vi "OSU_Sample.vi"() -> ()   [LabVIEW 2017]
uses:
  C:/Users/Ssantec_Test/Documents/Instrument_DLL_Sample_Labview_20220902_Ver1.2.2/DLL/x86/InstrumentDLL.dll
  DLL/x86/InstrumentDLL.dll
panel:
  in  "cmbdevname":u16(ring) caption="device name"
  in  "cmbosu_usb":u16(ring) caption="USB Resource"
  in  "txtPort":string caption="Port number(LAN)"
  in  "Address(GPIB、LAN)":string
  in  "OSU-110":T1(radio)
  in  "Target":enum32{"rdo100", "rdo110"}(radio)
  out "OSU":refnum<k24>
  in  "btn_Switch":bool
  in  "channel":u16(ring) items=["", "Ch1", "Ch2", "Ch3", "Ch4"]
  in  "Btn_DisConnect":bool
  in  "Btn_Connect":bool
  # "1. Connect"
  # "Communication"
  # "OSU-110"
  # "OSU-100"
  # "2. Setting function"
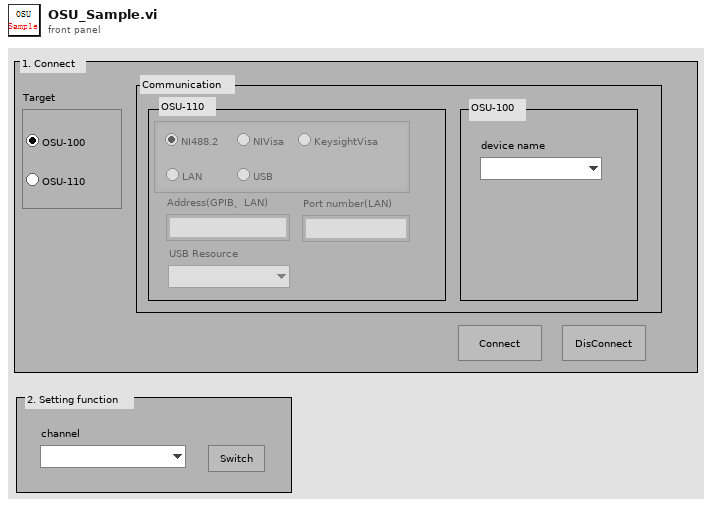
[diagram p1: front panel]
types:
  T1 = enum32{"rdiNI488", "rdiNIvisa", "rdikysightvisa", "rdoLAN", "rdiUSB"}
  T2 = enum8{"Enabled", "Disabled", "Disabled and Grayed Out"}
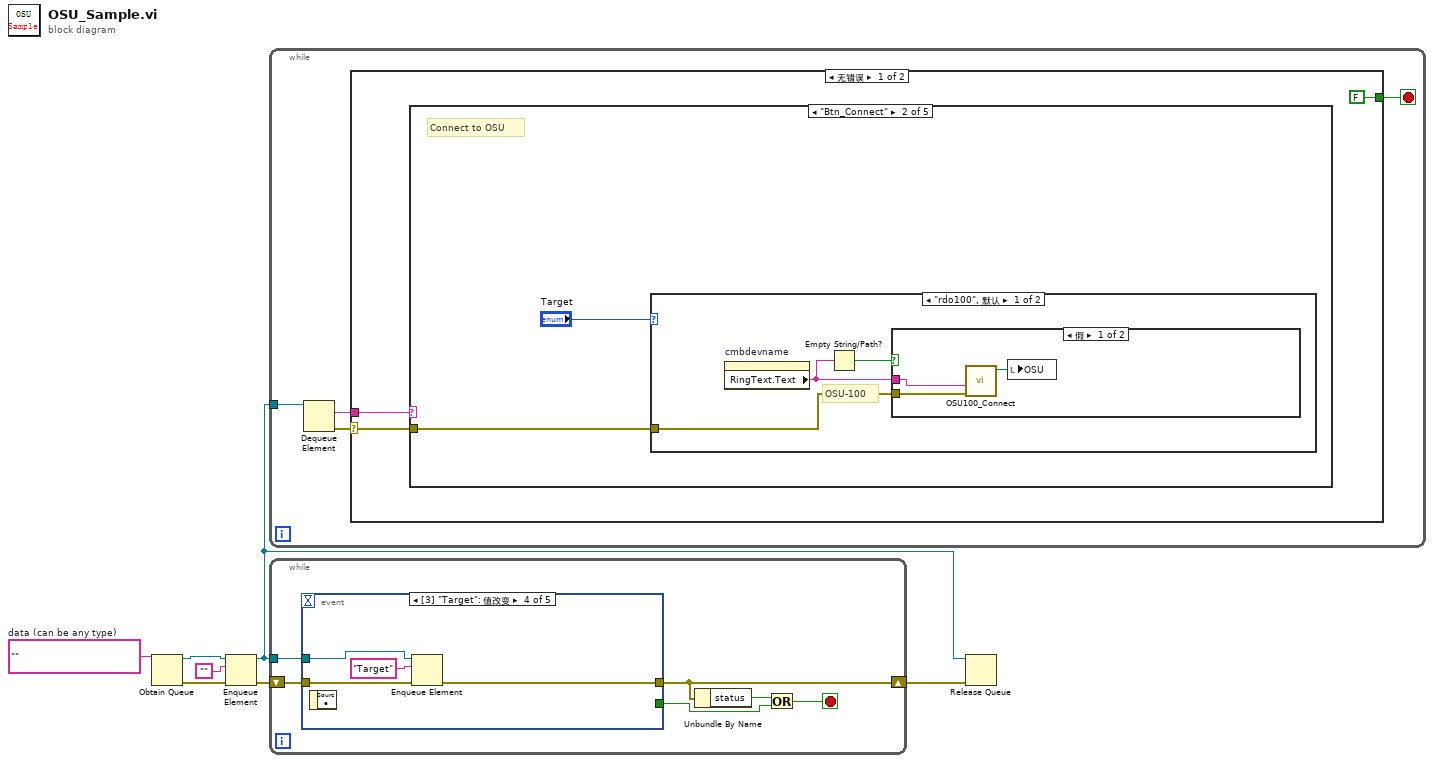
[diagram p0: block diagram]
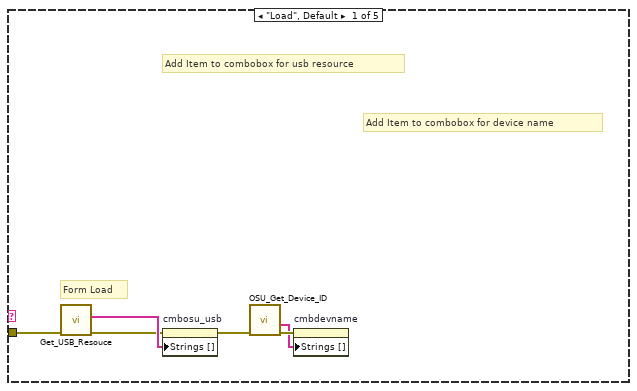
[diagram p2: hidden frame]
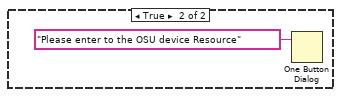
[diagram p3: hidden frame]
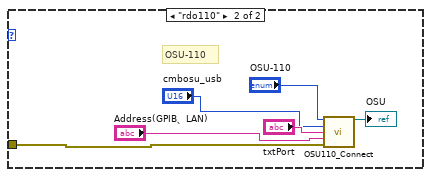
[diagram p4: hidden frame]
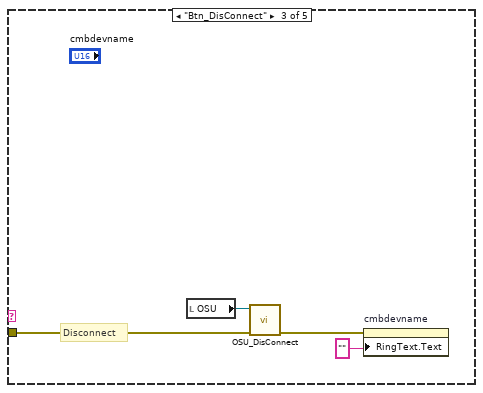
[diagram p5: hidden frame]
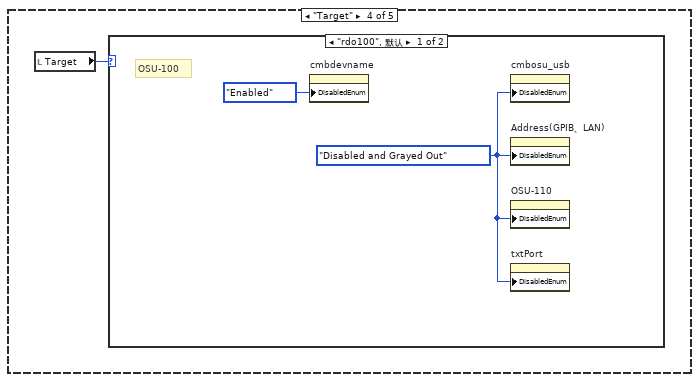
[diagram p6: hidden frame]
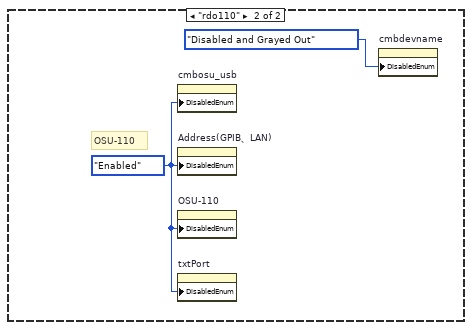
[diagram p7: hidden frame]
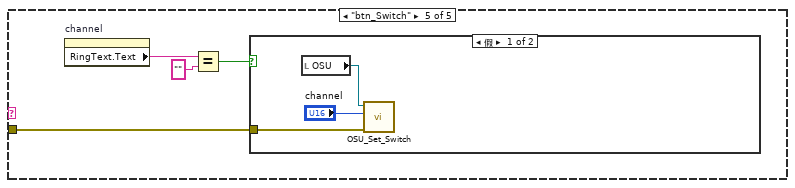
[diagram p8: hidden frame]
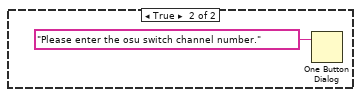
[diagram p9: hidden frame]
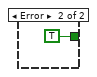
[diagram p10: hidden frame]
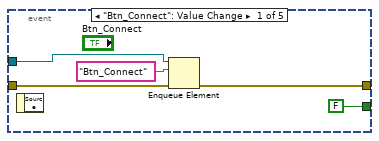
[diagram p11: hidden frame]
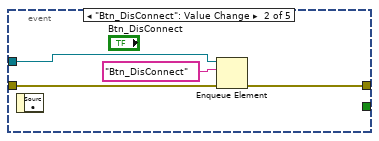
[diagram p12: hidden frame]
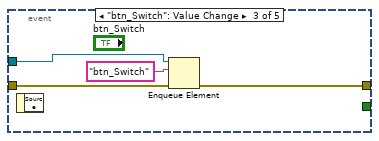
[diagram p13: hidden frame]
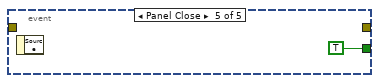
[diagram p14: hidden frame]
diagram:
  w6 = ""  # data (can be any type)
  n1 = Obtain Queue(element data type=w6) -> (queue out=w5:refnum<queue>, error out=w7:errorcluster)  [unwired: 4 in, 1 out]
  n2 = Enqueue Element(queue=w5, element="", error in (no error)=w7) -> (queue out=w1:refnum<queue>, error out=w3:errorcluster)  [unwired: 1 in, 1 out]
  n3 = while {
    tunnel: w1 -> [w11]
    stop <- w8 stop-if-true
    n4 = Dequeue Element(queue=w11) -> (element=w9:string, error out=w10:errorcluster)  [unwired: 2 in, 2 out]
    n5 = case shown="无错误" w10 {
      selector: w10 -> [w12 _]
      tunnel: w9 -> [w14 _]
      tunnel: [FALSE TRUE] -> w8
      frame No Error {
        n6 = case shown="\"Btn_Connect\"" w14 {
          tunnel: w12 -> [w20 w21 w38 _ w45]
          frame "Load", Default {
            # "Add Item to combobox for device name"
            # "Add Item to combobox for usb resource"
            # "Form Load"
            n7 = call "Get_USB_Resouce.vi"("error in (no error)"=w20) -> ("error out"=w18:errorcluster, "Get_USB_Resouce"=w19:string[])  [unwired: 8 in, 1 out]
            n8 = property on="cmbosu_usb" class="Ring (严格)"(error in=w18, "Strings []"=w19) -> (error out=w17:errorcluster)  [unwired: 1 in, 1 out]
            n9 = call "OSU_Get_Device_ID.vi"("error in (no error)"=w17) -> ("error out"=w16:errorcluster, "id"=w15:string[])  [unwired: 8 in, 1 out]
            n10 = property on="cmbdevname" class="Ring (严格)"(error in=w16, "Strings []"=w15) -> ()  [unwired: 1 in, 2 out]
          }
          frame "Btn_Connect" {
            # "Connect to OSU"
            n11 = case shown="\"rdo100\", 默认" "Target" {
              tunnel: w21 -> [w23 w31]
              frame "rdo100", Default {
                # "OSU-100"
                n12 = property on="cmbdevname" class="Ring (严格)"() -> ("RingText.Text"=w24:string)  [unwired: 2 in, 2 out]
                n13 = Empty String/Path?(string/path=w24) -> (empty?=w25:bool)
                n14 = case shown="假" w25 {
                  tunnel: w24 -> [w28 _]
                  tunnel: w23 -> [w27 _]
                  frame False {
                    n15 = call "OSU100_Connect.vi"("error in (no error)"=w27, "DeviceName"=w28) -> ("Reference out"=w26:refnum<k24>)  [unwired: 8 in, 1 out]
                    n16 = local write "OSU"(w26) -> ()
                  }
                  frame True {
                    n17 = One Button Dialog(message="Please enter to the OSU device Resource" ("消息")) -> ()  [unwired: 1 in, 1 out]
                  }
                }
              }
              frame "rdo110" {
                # "OSU-110"
                n18 = call "OSU110_Connect.vi"("OSU-110"="OSU-110", "cmbosu_usb"="cmbosu_usb", "txtPort"="txtPort", "DeviceName"="Address(GPIB、LAN)", "error in (no error)"=w31) -> ("Reference out"=→"OSU":refnum<k24>)  [unwired: 9 in, 1 out]
              }
            }
          }
          frame "Btn_DisConnect" {
            # "Disconnect"
            n19 = local read "OSU"() -> (w39:refnum<k24>)
            n20 = call "OSU_DisConnect.vi"("error in (no error)"=w38, ".NET Reference in"=w39) -> ("error out"=w36:errorcluster)  [unwired: 8 in, 1 out]
            n21 = property on="cmbdevname" class="Ring (严格)"(error in=w36, "RingText.Text"="" ("下拉列表文本.文本")) -> ()  [unwired: 1 in, 2 out]
          }
          frame "Target" {
            n22 = local read "Target"() -> (w40:enum32{"rdo100", "rdo110"})
            n23 = case shown="\"rdo100\", 默认" w40 {
              frame "rdo100", Default {
                w41 = T2."Disabled and Grayed Out" ("禁用")
                # "OSU-100"
                n24 = property on="cmbdevname" class="Ring (严格)"("DisabledEnum"=T2."Enabled" ("禁用")) -> ()  [unwired: 2 in, 2 out]
                n25 = property on="cmbosu_usb" class="Ring (严格)"("DisabledEnum"=w41) -> ()  [unwired: 2 in, 2 out]
                n26 = property on="Address(GPIB、LAN)" class="Str"("DisabledEnum"=w41) -> ()  [unwired: 2 in, 2 out]
                n27 = property on="OSU-110" class="RadioBtnsControl (严格)"("DisabledEnum"=w41) -> ()  [unwired: 2 in, 2 out]
                n28 = property on="txtPort" class="Str"("DisabledEnum"=w41) -> ()  [unwired: 2 in, 2 out]
              }
              frame "rdo110" {
                w43 = T2."Enabled" ("禁用")
                # "OSU-110"
                n29 = property on="cmbosu_usb" class="Ring (严格)"("DisabledEnum"=w43) -> ()  [unwired: 2 in, 2 out]
                n30 = property on="Address(GPIB、LAN)" class="Str"("DisabledEnum"=w43) -> ()  [unwired: 2 in, 2 out]
                n31 = property on="OSU-110" class="RadioBtnsControl (严格)"("DisabledEnum"=w43) -> ()  [unwired: 2 in, 2 out]
                n32 = property on="txtPort" class="Str"("DisabledEnum"=w43) -> ()  [unwired: 2 in, 2 out]
                n33 = property on="cmbdevname" class="Ring (严格)"("DisabledEnum"=T2."Disabled and Grayed Out" ("禁用")) -> ()  [unwired: 2 in, 2 out]
              }
            }
          }
          frame "btn_Switch" {
            n34 = property on="channel" class="Ring (严格)"() -> ("RingText.Text"=w48:string)  [unwired: 2 in, 2 out]
            n35 = Equal?(x=w48, y="") -> (x = y?=w46:bool)
            n36 = case shown="假" w46 {
              tunnel: w45 -> [w49 _]
              frame False {
                n37 = local read "OSU"() -> (w51:refnum<k24>)
                n38 = call "OSU_Set_Switch.vi"("error in (no error)"=w49, "channel"="channel", ".NET Reference in"=w51) -> ()  [unwired: 7 in, 2 out]
              }
              frame True {
                n39 = One Button Dialog(message="Please enter the osu switch channel number." ("消息")) -> ()  [unwired: 1 in, 1 out]
              }
            }
          }
        }
      }
      frame Error {
      }
    }
  }
  n40 = while {
    tunnel: w1 -> [w58]
    shift-right: [w56] -> w2
    shift-left: w3 -> [w57]
    stop <- w55 stop-if-true
    n41 = event shown="[3] \"Target\": 值改变" {
      selector: _ -> [_ _ _ _ _]
      dyn-events: _ -> [_ _ _ _ _]
      timeout: _ -> [_ _ _ _ _]
      tunnel: w58 -> [w64 w67 w72 w76 _]
      tunnel: w57 -> [w63 w66 w71 w75 _]
      tunnel: [w62 w65 w70 w74 _] -> w56
      tunnel: [FALSE ("y") _ _ _ TRUE ("y")] -> w54
      event "Btn_Connect": Value Change {
        n42 = event-data() -> ()  [unwired: 1 in, 1 out]
        n43 = Enqueue Element(queue=w64, element="Btn_Connect" ("元素"), error in (no error)=w63) -> (error out=w62:errorcluster)  [unwired: 1 in, 2 out]
      }
      event "Btn_DisConnect": Value Change {
        n44 = event-data() -> ()  [unwired: 1 in, 1 out]
        n45 = Enqueue Element(queue=w67, element="Btn_DisConnect" ("元素"), error in (no error)=w66) -> (error out=w65:errorcluster)  [unwired: 1 in, 2 out]
      }
      event "btn_Switch": Value Change {
        n46 = event-data() -> ()  [unwired: 1 in, 1 out]
        n47 = Enqueue Element(queue=w72, element="btn_Switch" ("元素"), error in (no error)=w71) -> (error out=w70:errorcluster)  [unwired: 1 in, 2 out]
      }
      event "Target": Value Change {
        n48 = event-data() -> ()  [unwired: 1 in, 1 out]
        n49 = Enqueue Element(queue=w76, element="Target" ("元素"), error in (no error)=w75) -> (error out=w74:errorcluster)  [unwired: 1 in, 2 out]
      }
      event Panel Close {
        n50 = event-data() -> ()  [unwired: 1 in, 1 out]
      }
    }
    n51 = Unbundle By Name(w56) -> ("status"=w59:bool)
    n52 = Or(x=w59, y=w54) -> (x .or. y?=w55:bool)
  }
  n53 = Release Queue(queue=w1, error in (no error)=w2) -> ()  [unwired: 1 in, 3 out]
